vi "Set Output Voltage.vi"(8 "error in (no error)":errorcluster, 10 "Voltage [V]":dbl, 11 "PSU In":refnum<class "DAQ.lvclass">) -> (0 "error out":errorcluster, 3 "PSU Out":refnum<class "DAQ.lvclass">)   [LabVIEW 2020, in "High Level PSU With Tests.lvlib" / "DAQ.lvclass"]
uses:
  DAQ.lvclass
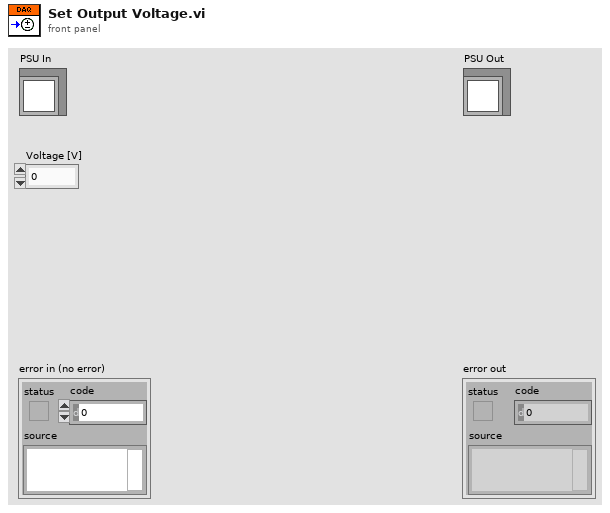
[diagram p1: front panel]
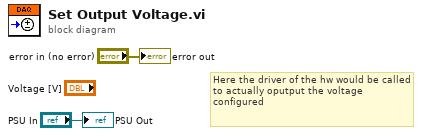
[diagram p0: block diagram]
diagram:
  # "Here the driver of the hw would be called to actually oputput the voltage configured"
  "error out" <- "error in (no error)"
  "PSU Out" <- "PSU In"
